vi "MQTT_Simple_Connect_and_Publish.vi"() -> ()   [LabVIEW 2025, in "DAQIO MQTT.lvlib"]
doc: "A simple client example that connects to a broker server and publishes messages to a topic.\n\n© 2015 - daq.io, LLC - Peter Adelhardt"
uses:
  DAQIO MQTT.lvlib
  Controls/Retain_Flag.ctl
  Controls/DUP_Flag.ctl
  Controls/Connection_Return_Codes.ctl
  Controls/Connect Flags.ctl
  Controls/User Info.ctl
panel:
  out "Message published":string
  in  "Stop Publishing":bool
  out "Message ID (acknowledged)":u16=10
  out "Acknowledged":bool
  in  "Message ID":u16=20
  in  "Message to be published":string="LabVIEW says it's "
  out "Connection Status":T1=enum."Connection refused: not authorized"
  out "error out":errorcluster
  in  "Client ID":string="LabVIEW_MQTT_Client"
  in  "error in (no error)":errorcluster
  in  "Topic":string="testtopic/LVMQTT"
  in  "Publish Meta":T4
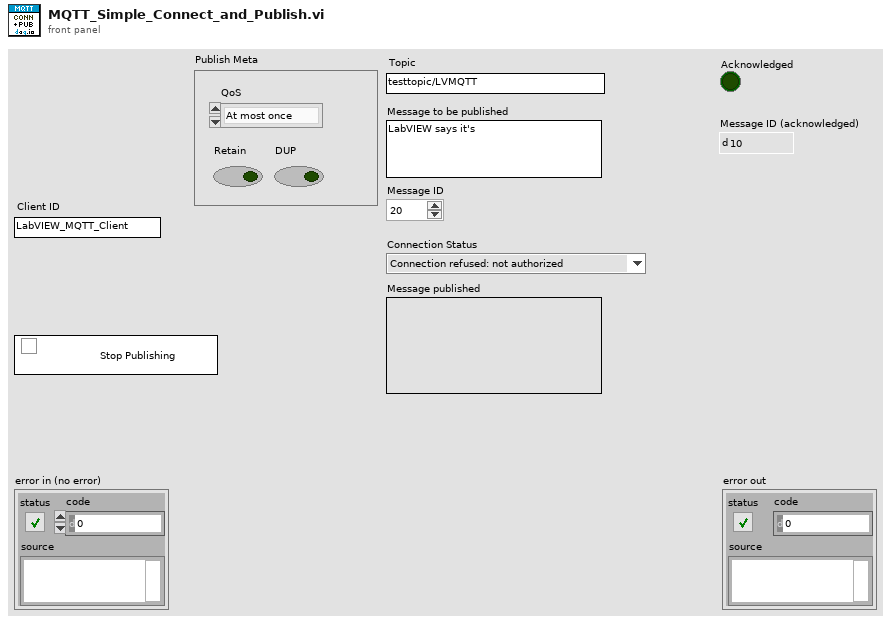
[diagram p1: front panel]
types:
  T1 = typedef "DAQIO MQTT.lvlib/Connection_Return_Codes.ctl" = enum16{"Connection accepted", "Connection refused: unacceptable protocol version", "Connection refused: identifier rejected", "Connection refused: Server unavailable", "Connection refused: bad user name or password", "Connection refused: not authorized"}
  T2 = typedef "DAQIO MQTT.lvlib/Retain_Flag.ctl" = bool
  T3 = typedef "DAQIO MQTT.lvlib/DUP_Flag.ctl" = bool
  T4 = cluster{"QoS":enum8{"At most once", "At least once", "Exactly once", "Reserved"}, "Retain":T2, "DUP":T3}
  T5 = typedef "DAQIO MQTT.lvlib/User Info.ctl" = cluster{"Username":string, "Password":string}
  T6 = typedef "DAQIO MQTT.lvlib/Connect Flags.ctl" = cluster{"user name":bool, "password":bool, "will retain":bool, "will flag":bool, "clean session":bool, "reserved":bool, "will QoS":enum8{"At most once", "At least once", "Exactly once", "Reserved"}}
  T7 = cluster{"QoS":enum8{"At most once", "At least once", "Exactly once", "Reserved"}, "DUP":T3, "Retain":T2, "Keep Alive (sec)":u16}
  T8 = enum8{"At most once", "At least once", "Exactly once", "Reserved"}
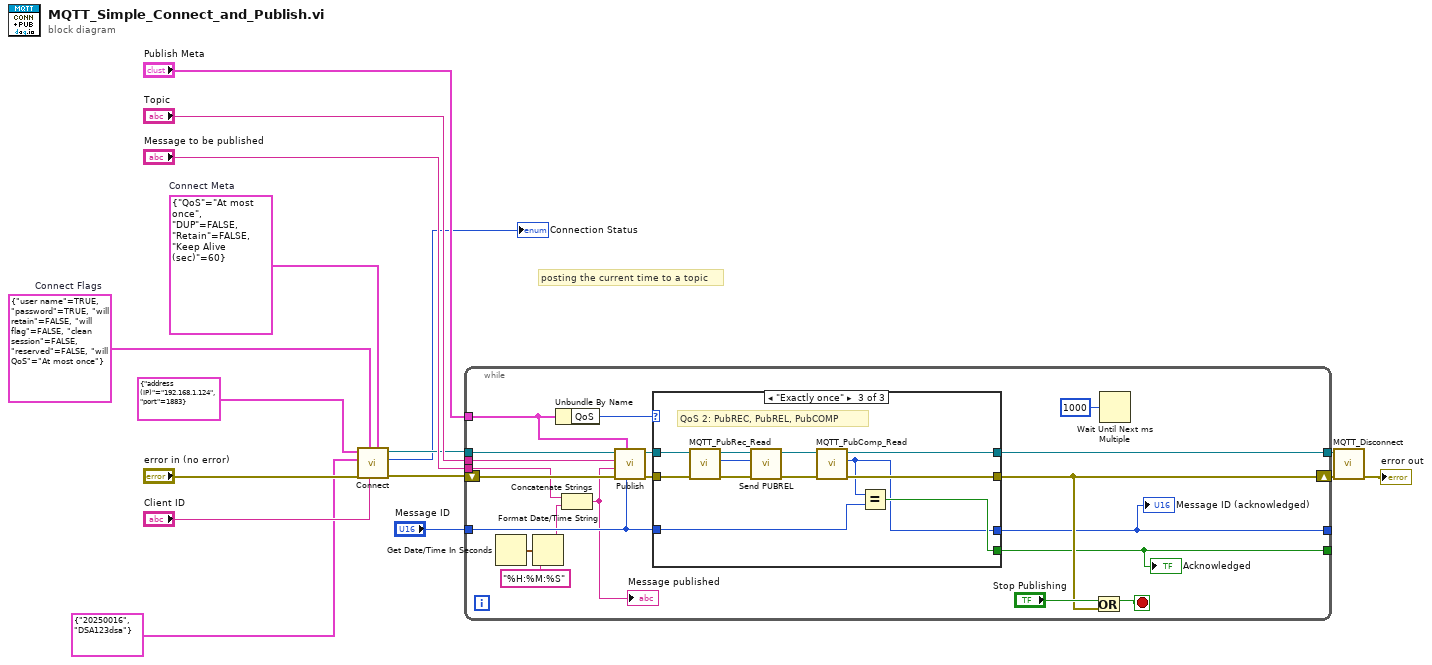
[diagram p0: block diagram]
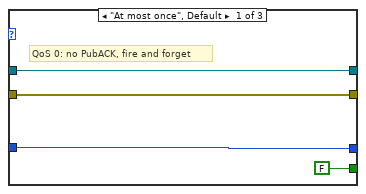
[diagram p2: hidden frame]
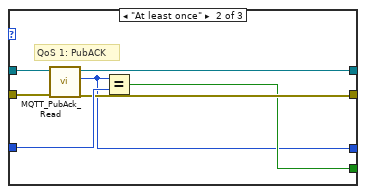
[diagram p3: hidden frame]
diagram:
  w14 = T6 {"user name"=TRUE, "password"=TRUE, "will retain"=FALSE, "will flag"=FALSE, "clean session"=FALSE, "reserved"=FALSE, "will QoS"=enum."At most once"}  # Connect Flags
  w11 = T7 {"QoS"=enum."At most once", "DUP"=FALSE, "Retain"=FALSE, "Keep Alive (sec)"=60}  # Connect Meta
  # "posting the current time to a topic"
  n1 = call "Connect.vi"("Connect Meta"=w11, "Client ID"="Client ID", "Connect Flags"=w14, "error in (no error)"="error in (no error)", "User Info"=T5 {"Username"="20250016", "Password"="DSA123dsa"}, "MQTT Broker"=cluster{"address (IP)":string, "port":u16} {"address (IP)"="192.168.1.124", "port"=1883}) -> ("error out"=w2:errorcluster, "Connection Status"=→"Connection Status":T1, "connection ID out"=w4:refnum<k5>)  [unwired: 3 in]
  n2 = while {
    tunnel: "Topic" -> [w36]
    tunnel: "Message to be published" -> [w26]
    tunnel: w4 -> [w35]
    tunnel: "Publish Meta" -> [w33]
    tunnel: [w29] -> w7
    tunnel: "Message ID" -> [w28]
    tunnel: [w18] -> _
    tunnel: [w17] -> _
    shift-right: [w20] -> w8
    shift-left: w2 -> [w34]
    stop <- w21 stop-if-true
    n3 = Get Date/Time In Seconds() -> (seconds since 1Jan1904=w25:timestamp)
    n4 = Format Date/Time String(time format string (%c)="%H:%M:%S", seconds (now)=w25) -> (date/time string=w23:string)  [unwired: 1 in]
    n5 = Unbundle By Name(w33) -> ("QoS"=w32:T8)
    n6 = Concatenate Strings(w26, w23) -> (w22:string)
    "Message published" <- w22
    n7 = call "Publish.vi"("Message ID"=w28, "Publish Meta"=w33, "error in (no error)"=w34, "Message to be published"=w22, "Topic"=w36, "connection ID"=w35) -> ("error out"=w31:errorcluster, "connection ID out"=w30:refnum<k5>)  [unwired: 4 in]
    n8 = case shown="\"Exactly once\"" w32 {
      tunnel: w31 -> [w39 w46 w58]
      tunnel: w30 -> [w40 w47 w59]
      tunnel: [w39 w44 w51] -> w20
      tunnel: [w40 w43 w52] -> w29
      tunnel: w28 -> [w37 w45 w57]
      tunnel: [FALSE w42 w53] -> w18
      tunnel: [w37 w41 w50] -> w17
      frame "At most once", Default {
        # "QoS 0: no PubACK, fire and forget"
      }
      frame "At least once" {
        # "QoS 1: PubACK"
        n9 = call "MQTT_PubAck_Read.vi"("error in (no error)"=w46, "connection ID"=w47) -> ("error out"=w44:errorcluster, "Message ID"=w41:u16, "connection ID out"=w43:refnum<k5>)  [unwired: 7 in]
        n10 = Equal?(x=w41, y=w45) -> (x = y?=w42:bool)
      }
      frame "Exactly once" {
        # "QoS 2: PubREC, PubREL, PubCOMP"
        n11 = call "MQTT_PubRec_Read.vi"("error in (no error)"=w58, "connection ID"=w59) -> ("error out"=w56:errorcluster, "Message ID"=w54:u16, "connection ID out"=w55:refnum<k5>)  [unwired: 7 in]
        n12 = call "Send PUBREL.vi"("error in (no error)"=w56, "Message ID"=w54, "connection ID"=w55) -> ("error out"=w48:errorcluster, "connection ID out"=w49:refnum<k5>)  [unwired: 7 in]
        n13 = call "MQTT_PubComp_Read.vi"("error in (no error)"=w48, "connection ID"=w49) -> ("error out"=w51:errorcluster, "Message ID"=w50:u16, "connection ID out"=w52:refnum<k5>)  [unwired: 7 in]
        n14 = Equal?(x=w50, y=w57) -> (x = y?=w53:bool)
      }
    }
    "Message ID (acknowledged)" <- w17
    "Acknowledged" <- w18
    n15 = Or(x="Stop Publishing", y=w20) -> (x .or. y?=w21:bool)
    n16 = Wait Until Next ms Multiple(millisecond multiple=u32 1000) -> ()  [unwired: 1 out]
  }
  n17 = call "MQTT_Disconnect.vi"("error in (no error)"=w8, "connection ID"=w7) -> ("error out"=→"error out":errorcluster)  [unwired: 9 in]
